vi "Init Condition.vi"(5 "Sequencing":refnum<class "MessageQ.lvclass">, 6 "Variables":refnum<class "Variables.lvclass">, 7 "VolatusAPI":refnum<class "VolatusAPI.lvclass">, 8 "error in (no error)":refnum<class "MultiErrors.lvclass">, 10 "Condition Config":refnum<class "Condition Config.lvclass">, 11 "Time Condition in":refnum<class "Time Condition.lvclass">) -> (0 "error out":refnum<class "MultiErrors.lvclass">, 3 "Time Condition out":refnum<class "Time Condition.lvclass">)   [LabVIEW 2020, in "VolatusSeq.lvlib" / "Time Condition.lvclass"]
uses:
  Time Condition.lvclass
  VolatusErrorUtilities/MultiErrors/MultiErrors.lvclass
  Volatus/VolatusAPI/VolatusAPI.lvclass
  VolatusSeqConfig/Condition Config/Condition Config.lvclass
  Volatus/MessageQ/MessageQ.lvclass
  VolatusSeqConfig/Time Condition Config/Time Condition Config.lvclass
  VolatusSeqConfig/Time Condition Config/Time Condition Config.lvclass/Time Condition Config.ctl
  Time Condition.lvclass/Time Condition.ctl
  Variables/Variables.lvclass
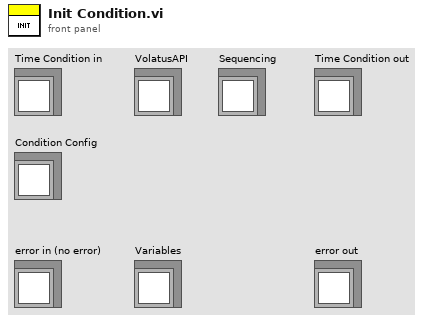
[diagram p1: front panel]
types:
  T1 = typedef "VolatusSeqConfig.lvlib/Timer.ctl" = enum16{"Sequence", "State", "Wall"}
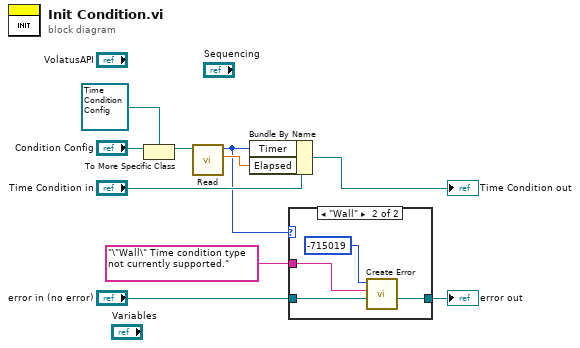
[diagram p0: block diagram]
diagram:
  n1 = To More Specific Class(target class=refnum<class "Time Condition Config.lvclass"> refnum ("VolatusSeqConfig.lvlib:Time Condition Config.lvclass"), reference="Condition Config") -> (specific class reference=w7:refnum<class "Time Condition Config.lvclass">)  [unwired: 1 in, 1 out]
  n2 = call "Read.vi"("Time Condition Config in"=w7) -> ("Elapsed"=w5:dbl, "Timer"=w4:T1)  [unwired: 9 in]
  n3 = Bundle By Name(cluster="Time Condition in", "Timer"=w4, "Elapsed"=w5) -> (→"Time Condition out":refnum<class "Time Condition.lvclass">)
  n4 = case shown="\"Wall\"" w4 {
    tunnel: "\"Wall\" Time condition type not currently supported." -> [_ w14]
    tunnel: "error in (no error)" -> [w11 w13]
    tunnel: [w11 w12] -> w1
    frame Default {
    }
    frame "Wall" {
      n5 = call "Create Error.vi"("MultiErrors in"=w13, "Message"=w14, "Code"=-715019 ("error code (0)")) -> ("MultiErrors out"=w12:refnum<class "MultiErrors.lvclass">)  [unwired: 8 in]
    }
  }
  "error out" <- w1
